vi "Logger Programatic Entry.vi"(0 "Log File Input":T1, 11 "error in (no error)":errorcluster) -> (15 "error out":errorcluster)   [LabVIEW 2018]
uses:
  Log File Input.ctl
  Logger Global.vi
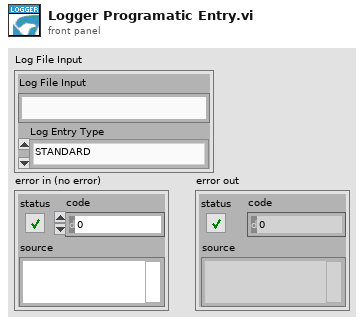
[diagram p1: front panel]
types:
  T1 = typedef "Log File Input.ctl" = cluster{"Log File Input":string, "Log Entry Type":enum16{"STANDARD", "WARNING", "CRITICAL"}}
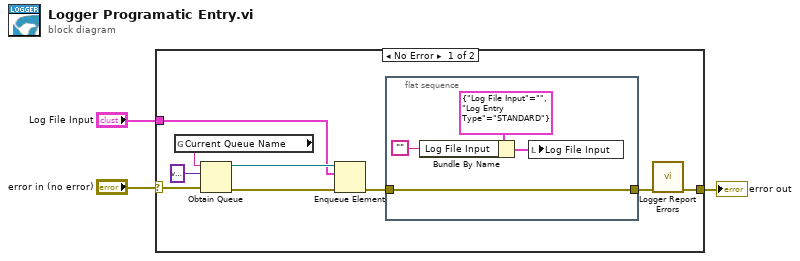
[diagram p0: block diagram]
diagram:
  n1 = case shown="No Error" "error in (no error)" {
    selector: "error in (no error)" -> [w12 w17]
    tunnel: [w4 w17] -> w1
    tunnel: "Log File Input" -> [w6 _]
    frame No Error {
      n2 = global read "Logger Global.vi" "Current Queue Name"() -> (w9:string)
      n3 = Obtain Queue(name (unnamed)=w9, element data type=variant, error in (no error)=w12) -> (queue out=w10:refnum<queue>, error out=w11:errorcluster)  [unwired: 2 in, 1 out]
      n4 = Enqueue Element(queue=w10, element=w6, error in (no error)=w11) -> (error out=w7:errorcluster)  [unwired: 1 in, 2 out]
      n5 = flat-sequence {
        tunnel: [w16] -> w5
        tunnel: w7 -> [w16]
        frame #0 {
          n6 = Bundle By Name(cluster=T1 {"Log File Input"="", "Log Entry Type"=enum."STANDARD"} ("Log File Input"), "Log File Input"="") -> (w15:T1)
          n7 = local write "Log File Input"(w15) -> ()
        }
      }
      n8 = call "Logger Report Errors.vi"("error in (no error)"=w5) -> ("error out"=w4:errorcluster)  [unwired: 14 in]
    }
    frame Error {
    }
  }
  "error out" <- w1
